vi "Select Files.vi"(6 "Same Desc":bool, 7 "Desc in":string[](array[string]), 8 "error in (no error)":errorcluster, 9 "Select FP Item In":T1, 10 "All / Selected by Name":bool, 11 "VI in":refnum<vi>) -> (0 "error out":errorcluster, 1 "Select FP Item Out":T1, 3 "Desc out":string[](array[string]))   [LabVIEW 2020]
uses:
  TDefs/Selected FP Items.ctl
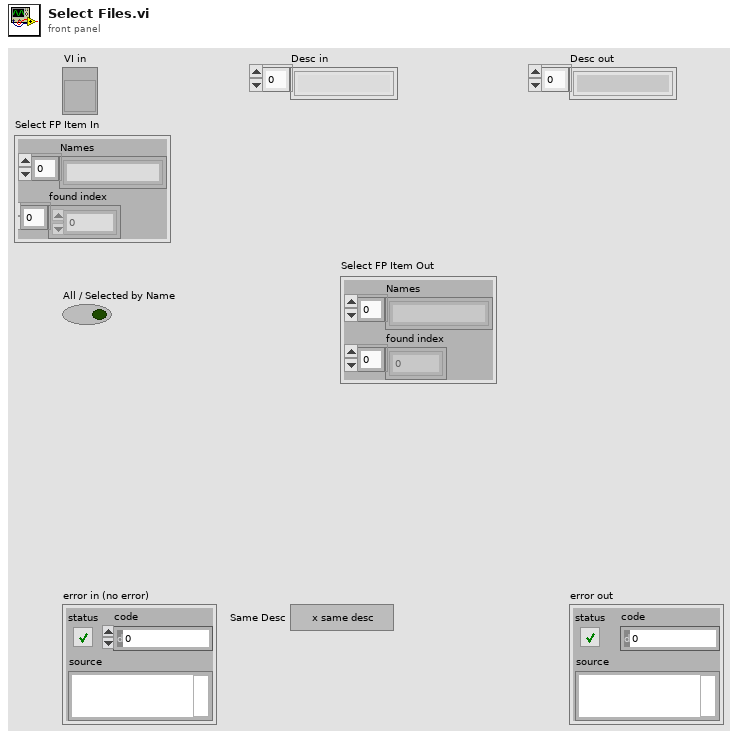
[diagram p1: front panel]
types:
  T1 = typedef "Selected FP Items.ctl" = cluster{"Names":string[], "found index":i32[]}
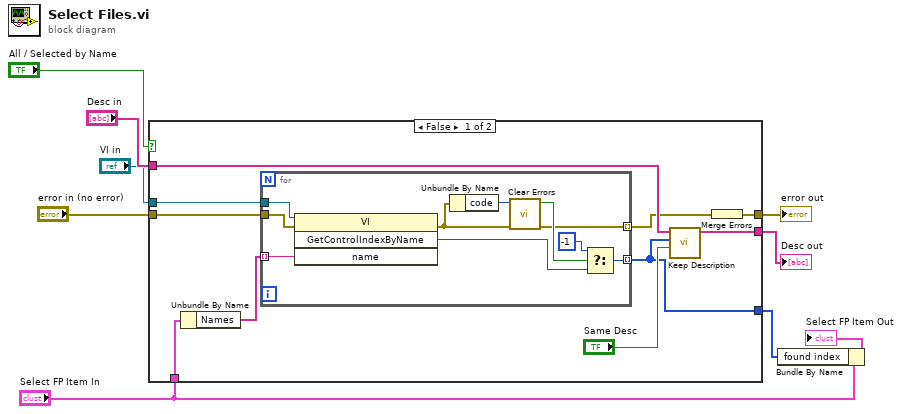
[diagram p0: block diagram]
diagram:
  n1 = case shown="False" "All / Selected by Name" {
    tunnel: "VI in" -> [w19 _]
    tunnel: "Desc in" -> [w18 w31]
    tunnel: [w16 w31] -> w7
    tunnel: [w15 _] -> w1
    tunnel: "error in (no error)" -> [w14 w30]
    tunnel: [w12 w30] -> w9
    tunnel: "Select FP Item In" -> [w11 _]
    frame False {
      n2 = Unbundle By Name(w11) -> ("Names"=w10:string[])
      n3 = for {
        tunnel: w19 -> [w29]
        tunnel: w10 -> [w23] mode=indexing
        tunnel: [w22] -> w15 mode=indexing
        tunnel: w14 -> [w21]
        tunnel: [w20] -> w13 mode=indexing
        n4 = invoke class="VI" method="GetControlIndexByName"(reference=w29, error in=w21, "name"=w23) -> (error out=w28:errorcluster, "GetControlIndexByName"=w25:i32)  [unwired: 1 in, 2 out]
        n5 = Unbundle By Name(w28) -> ("code"=w27:i32)
        n6 = call <vilib>:"Clear Errors.vi"("error in (no error)"=w28, "specific error code to clear (0: all)"=w27) -> ("error out"=w20:errorcluster, "specific error cleared?"=w26:bool)  [unwired: 4 in]
        n7 = Select(t=-1, s=w26, f=w25) -> (s? t:f=w22:i32)
      }
      n8 = call "Keep Description.vi"("Same Desc"="Same Desc", "Array"=w15, "Value in"=w18) -> ("Value out"=w16:string[])  [unwired: 8 in]
      n9 = Merge Errors(w13) -> (w12:errorcluster)
    }
    frame True {
    }
  }
  "error out" <- w9
  "Desc out" <- w7
  n10 = Bundle By Name(cluster="Select FP Item In", "found index"=w1) -> (→"Select FP Item Out":T1)
